vi "LakeShore218_close.vi"(8 "error in":errorcluster, 11 "VISA in":refnum<visa-resource-name>) -> (0 "error out":errorcluster)   [LabVIEW 2019]
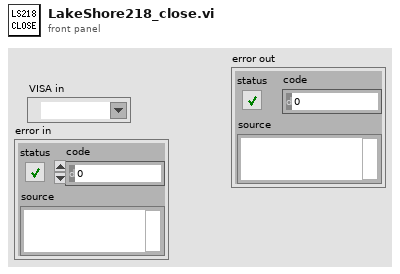
[diagram p1: front panel]
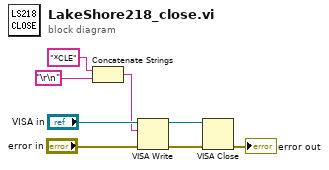
[diagram p0: block diagram]
diagram:
  n1 = Concatenate Strings("*CLE" ("write buffer 2"), "\r\n") -> (w6:string)
  n2 = VISA Write(VISA resource name="VISA in", write buffer=w6, error in (no error)="error in") -> (VISA resource name out=w8:refnum<visa-resource-name>, error out=w2:errorcluster)  [unwired: 1 out]
  n3 = VISA Close(VISA resource name=w8, error in (no error)=w2) -> (error out=→"error out":errorcluster)
